vi "ToInt16.vi"(1 "index":i32, 2 "array":u8[](array[numeric])) -> (0 "sp float":i16)   [LabVIEW 2009]
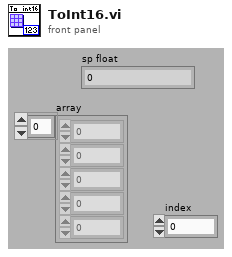
[diagram p1: front panel]
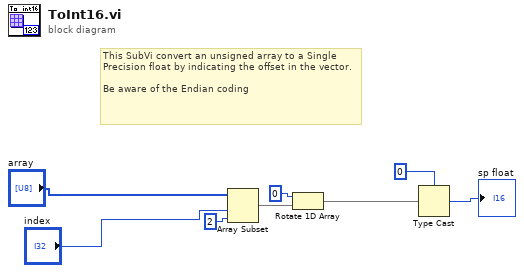
[diagram p0: block diagram]
diagram:
  # "This SubVi convert an unsigned array to a Single Precision float by indicating the offset in the vector.\n\nBe aware of the Endian coding"
  n1 = Array Subset(array="array", index="index", length=2) -> (w5:u8[])
  n2 = Rotate 1D Array(1:w5, 2:0 ("n")) -> (0:w1:u8[])
  n3 = Type Cast(type=i16 0 ("sp float"), x=w1) -> (*(type *) &x=→"sp float":i16)
